vi "CLD 12 Sequencer State Machine solution 2.vi"() -> ()   [LabVIEW 2019]
doc: "CLD 12: Sequences boolean values in the order they are loaded from the file."
uses:
  Controls/CLD 12 Data Cluster.ctl
  Controls/CLD 12 Sequencer Enum.ctl
  CLD3 Timer/CLD3 FGV Mode.ctl
panel:
  out "Current Time Target":dbl
  in  "error in (no error)":errorcluster
  out "error out":errorcluster
  in  "Stop Button":bool
  out "Time Elapsed":dbl
  out "Switch 3":bool
  out "Switch 2":bool
  out "Switch 1":bool
  in  "Start":bool
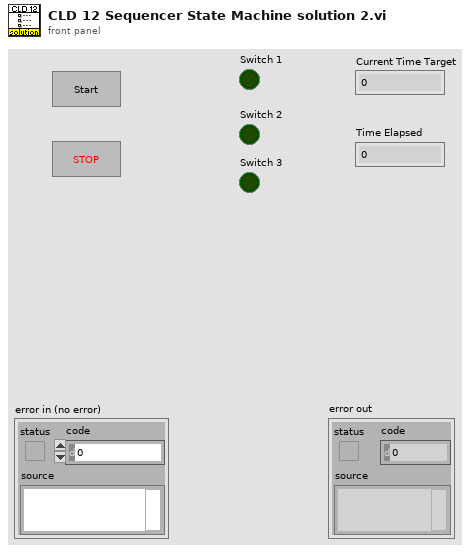
[diagram p1: front panel]
types:
  T1 = typedef "CLD 12 Data Cluster.ctl" = cluster{"Command":T2, "Time Value":dbl, "Boolean":bool, "Boolean 2":bool, "Boolean 3":bool}
  T2 = typedef "CLD 12 Sequencer Enum.ctl" = enum16{"Initialize", "SetTime", "RunState1", "Runstate2", "Idle", "Start"}
  T3 = typedef "CLD3 FGV Mode.ctl" = enum16{"Start Timer", "Reset Timer", "Read Time", "Pause", "Resume"}
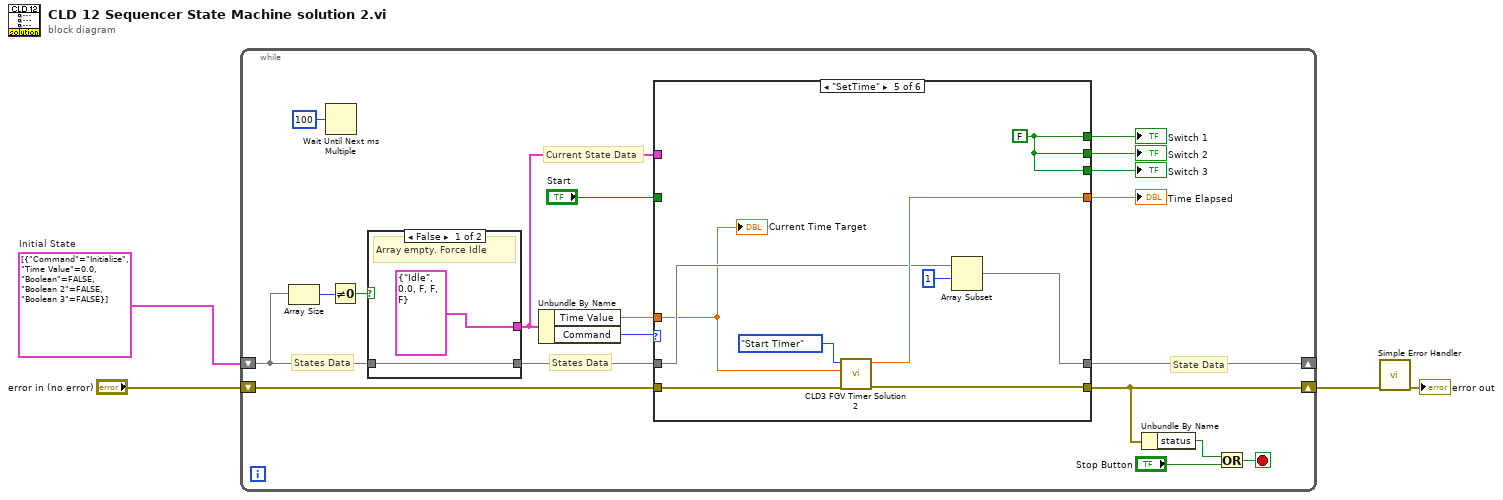
[diagram p0: block diagram]
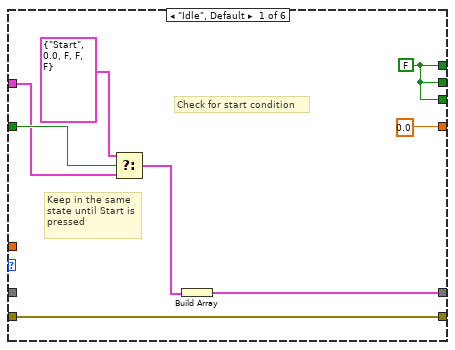
[diagram p2: hidden frame]
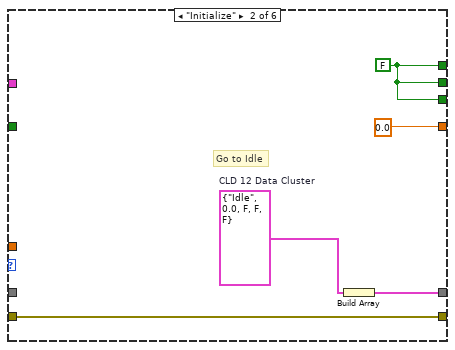
[diagram p3: hidden frame]
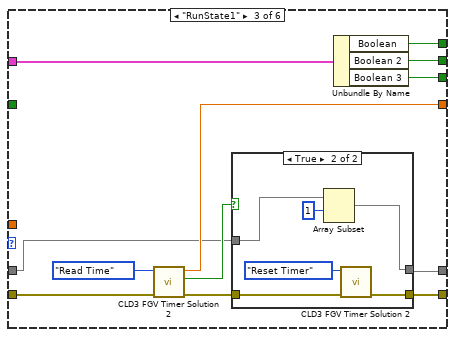
[diagram p4: hidden frame]
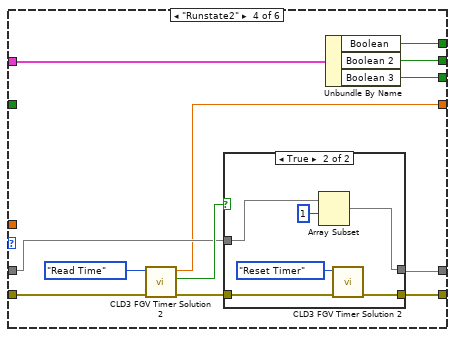
[diagram p6: hidden frame]
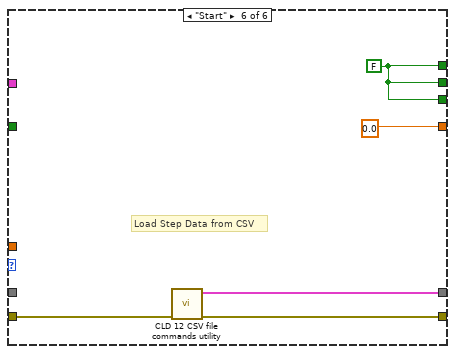
[diagram p8: hidden frame]
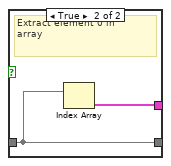
[diagram p9: hidden frame]
diagram:
  w1 = T1[] [{"Command"=enum."Initialize", "Time Value"=0.0, "Boolean"=FALSE, "Boolean 2"=FALSE, "Boolean 3"=FALSE}]  # Initial State
  n1 = while {
    shift-right: [w21] -> w2
    shift-left: "error in (no error)" -> [w19]
    shift-right: [w5] -> _
    shift-left: w1 -> [w11]
    stop <- w22 stop-if-true
    # "Current State Data"
    # "States Data"
    # "State Data"
    # "States Data"
    n2 = Array Size(array=w11) -> (size(s)=w10:i32)
    n3 = Wait Until Next ms Multiple(millisecond multiple=u32 100) -> ()  [unwired: 1 out]
    n4 = Not Equal To 0?(x=w10) -> (x != 0?=w9:bool)
    n5 = case shown="False" w9 {
      tunnel: [T1 {"Command"=enum."Idle", "Time Value"=0.0, "Boolean"=FALSE, "Boolean 2"=FALSE, "Boolean 3"=FALSE} ("CLD 12 Data Cluster") w94] -> w13
      tunnel: w11 -> [w91 w93]
      tunnel: [w91 w93] -> w8
      frame False {
        # "Array empty. Force Idle"
      }
      frame True {
        # "Extract element 0 in \narray"
        n6 = Index Array(array=w93) -> (element=w94:T1)  [unwired: 1 in]
      }
    }
    n7 = Unbundle By Name(w13) -> ("Time Value"=w12:dbl, "Command"=w14:T2)
    n8 = case shown="\"SetTime\"" w14 {
      tunnel: [w28 w36 w40 w65 w83 w89] -> w21
      tunnel: w19 -> [w28 w36 w47 w62 w84 w90]
      tunnel: [w31 w35 w45 w59 w85 w88] -> w18
      tunnel: [w31 w35 w44 w58 w85 w88] -> w17
      tunnel: [w31 w35 w43 w57 w85 w88] -> w16
      tunnel: [0.0 ("Elapsed Time (s.ss)") 0.0 ("Elapsed Time (s.ss)") w46 w60 w81 0.0 ("Elapsed Time (s.ss)")] -> w15
      tunnel: [w29 w34 w38 w64 w78 w87] -> w5
      tunnel: w13 -> [w26 _ w37 w61 _ _]
      tunnel: w12 -> [_ _ _ _ w77 _]
      tunnel: w8 -> [_ _ w39 w63 w79 _]
      tunnel: "Start" -> [w27 _ _ _ _ _]
      frame "Idle", Default {
        w31 = FALSE ("Boolean 1")
        # "Keep in the same \nstate until Start is \npressed"
        # "Check for start condition"
        n9 = Select(t=T1 {"Command"=enum."Start", "Time Value"=0.0, "Boolean"=FALSE, "Boolean 2"=FALSE, "Boolean 3"=FALSE}, s=w27, f=w26) -> (s? t:f=w25:T1)
        n10 = Build Array(w25) -> (w29:T1[])
      }
      frame "Initialize" {
        w35 = FALSE ("Boolean 1")
        w32 = T1 {"Command"=enum."Idle", "Time Value"=0.0, "Boolean"=FALSE, "Boolean 2"=FALSE, "Boolean 3"=FALSE}  # CLD 12 Data Cluster
        # "Go to Idle"
        n11 = Build Array(w32) -> (w34:T1[])
      }
      frame "RunState1" {
        n12 = call "CLD3 FGV Timer Solution 2.vi"("Error In"=w47, "Timer Mode"=CLD3_FGV_Mode."Read Time") -> ("Error Out"=w41:errorcluster, "Has Time Elapsed"=w42:bool, "Elapsed Time (s.ss)"=w46:dbl)  [unwired: 7 in]
        n13 = case shown="True" w42 {
          tunnel: w41 -> [w49 w56]
          tunnel: [w49 w55] -> w40
          tunnel: w39 -> [w50 w53]
          tunnel: [w50 w51] -> w38
          frame False {
          }
          frame True {
            n14 = Array Subset "Array Subset"(array=w53, index=1) -> (w51:T1[])  [unwired: 1 in]
            n15 = call "CLD3 FGV Timer Solution 2.vi"("Error In"=w56, "Timer Mode"=CLD3_FGV_Mode."Reset Timer") -> ("Error Out"=w55:errorcluster)  [unwired: 7 in, 2 out]
          }
        }
        n16 = Unbundle By Name(w37) -> ("Boolean"=w45:bool, "Boolean 2"=w44:bool, "Boolean 3"=w43:bool)
      }
      frame "Runstate2" {
        n17 = call "CLD3 FGV Timer Solution 2.vi"("Error In"=w62, "Timer Mode"=CLD3_FGV_Mode."Read Time") -> ("Error Out"=w66:errorcluster, "Has Time Elapsed"=w67:bool, "Elapsed Time (s.ss)"=w60:dbl)  [unwired: 7 in]
        n18 = case shown="True" w67 {
          tunnel: w66 -> [w69 w76]
          tunnel: [w69 w75] -> w65
          tunnel: w63 -> [w70 w73]
          tunnel: [w70 w71] -> w64
          frame False {
          }
          frame True {
            n19 = Array Subset "Array Subset"(array=w73, index=1) -> (w71:T1[])  [unwired: 1 in]
            n20 = call "CLD3 FGV Timer Solution 2.vi"("Error In"=w76, "Timer Mode"=CLD3_FGV_Mode."Reset Timer") -> ("Error Out"=w75:errorcluster)  [unwired: 7 in, 2 out]
          }
        }
        n21 = Unbundle By Name(w61) -> ("Boolean"=w59:bool, "Boolean 2"=w58:bool, "Boolean 3"=w57:bool)
      }
      frame "SetTime" {
        w85 = FALSE ("Boolean 1")
        n22 = call "CLD3 FGV Timer Solution 2.vi"("Error In"=w84, "Time Target (s)"=w77, "Timer Mode"=CLD3_FGV_Mode."Start Timer") -> ("Error Out"=w83:errorcluster, "Elapsed Time (s.ss)"=w81:dbl)  [unwired: 6 in, 1 out]
        n23 = Array Subset "Array Subset"(array=w79, index=1) -> (w78:T1[])  [unwired: 1 in]
        "Current Time Target" <- w77
      }
      frame "Start" {
        w88 = FALSE ("Boolean 1")
        # "Load Step Data from CSV"
        n24 = call "CLD 12 CSV file commands utility.vi"("Error In"=w90) -> ("Error Out"=w89:errorcluster, "Command Array Out"=w87:T1[])  [unwired: 9 in]
      }
    }
    "Time Elapsed" <- w15
    "Switch 1" <- w18
    "Switch 2" <- w17
    "Switch 3" <- w16
    n25 = Unbundle By Name(w21) -> ("status"=w20:bool)
    n26 = Or(x=w20, y="Stop Button") -> (x .or. y?=w22:bool)
  }
  n27 = call <vilib>:"Simple Error Handler.vi"("error in (no error)"=w2) -> ("error out"=→"error out":errorcluster)  [unwired: 4 in, 4 out]
